vi "PM100D_Ranging.vi"(0 "VISA in":refnum<visa-resource-name>="USB0::0x1313::0x8070::P0000118::INSTR", 7 "Index":i16 min=0 max=5 step=1, 9 "AUTO":bool, 11 "error in (no error)":errorcluster, 12 "Unit":string(combo)="POW") -> (1 "SensType":i32(ring) items=["No Sensor", "Photo", "Thermo", "Pyro"], 3 "AUTO?":bool, 4 "VISA out":refnum<visa-resource-name>, 5 "AutoOut":bool, 6 "RANG_Val":dbl, 10 "RANG_lbl":string, 14 "IndexOut":i32, 15 "error out":errorcluster)   [LabVIEW 2015]
panel:
  out "Rng_Array":string[](array[string])
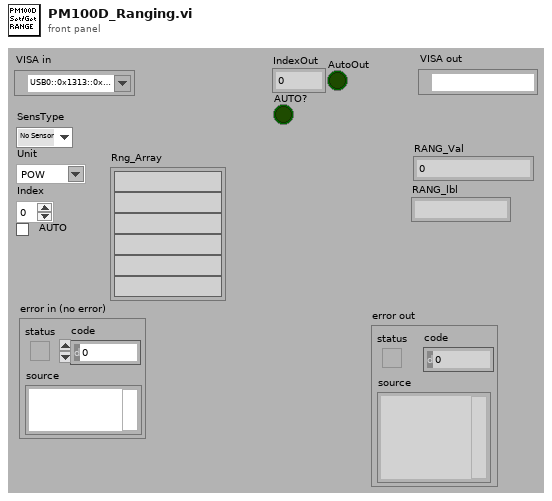
[diagram p1: front panel]
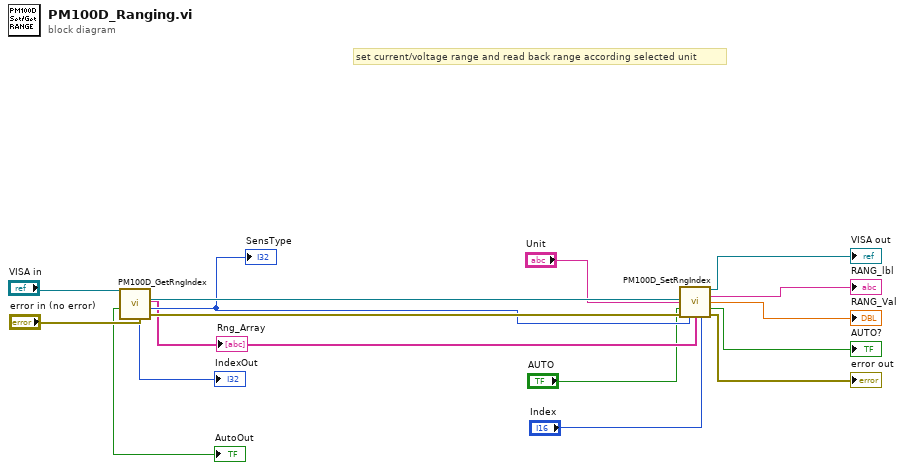
[diagram p0: block diagram]
diagram:
  # "set current/voltage range and read back range according selected unit"
  n1 = call "PM100D_GetRngIndex.vi"("error in (no error)"="error in (no error)", "VISA in"="VISA in") -> ("error out"=w11:errorcluster, "SensType"=w6:i32, "Rng_Array"=w3:string[], "dup VISA session"=w12:refnum<visa-resource-name>, "IndexOut"=→"IndexOut":i32, "AutoOut"=→"AutoOut":bool)  [unwired: 4 in]
  "SensType" <- w6
  "Rng_Array" <- w3
  n2 = call "PM100D_SetRngIndex.vi"("VISAin"=w12, "Unit"="Unit", "AUTO"="AUTO", "error in"=w11, "SensType"=w6, "Rng_Array"=w3, "Index"="Index") -> ("VISAout"=→"VISA out":refnum<visa-resource-name>, "lblRange"=→"RANG_lbl":string, "Numeric 2"=→"RANG_Val":dbl, "AUTO?"=→"AUTO?":bool, "error out 2"=→"error out":errorcluster)  [unwired: 4 in]
